vi "Destroy Broadcast Events.vi"(8 "error in (no error)":errorcluster) -> (0 "error out":errorcluster)   [LabVIEW 2015, in "Tool Module.lvlib"]
doc: "Destroy the broadcast events, even if there is an incoming error.\n\n<b>NOTE</b>: The contents of this VI are automatically generated and modified by the <b>Tools > Delacor > DQMH</b> utilities. Consider using those utilities instead of making your own modifications to this VI.\n_____\nBased on Delacor QMH Project Template 2.1.0.2."
uses:
  Tool Module.lvlib
panel:
  # "NOTE: The contents of this VI are automatically generated and modified by the Tools > Delacor > DQMH utilities. Consider using those utilities instead of making your own modifications to this VI."
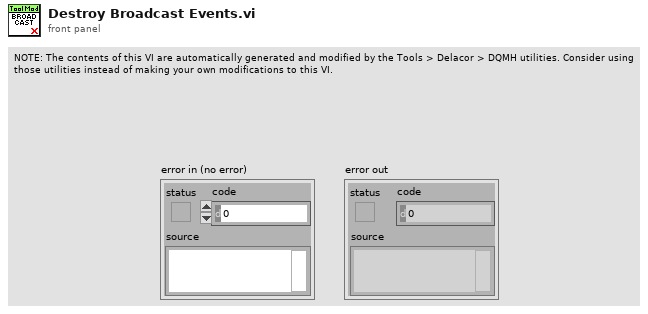
[diagram p1: front panel]
types:
  T1 = typedef "Tool Module.lvlib/Broadcast Events--cluster.ctl" = cluster{"Module Did Init":refnum<user-event>, "Status Updated":refnum<user-event>, "Error Reported":refnum<user-event>, "Module Did Stop":refnum<user-event>, "Update Module Execution Status":refnum<user-event>, "Send Status":refnum<user-event>, "Trigger":refnum<user-event>, "Connected":refnum<user-event>, "Read from File Rtn":refnum<user-event>, "Device Temperature":refnum<user-event>}
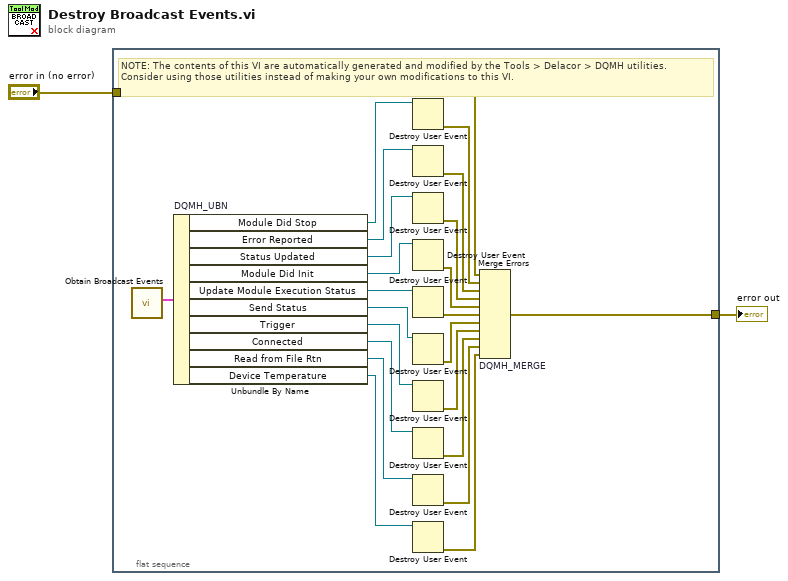
[diagram p0: block diagram]
diagram:
  n1 = flat-sequence {
    tunnel: [w24] -> w2
    tunnel: "error in (no error)" -> [w15]
    frame #0 {
      # "NOTE: The contents of this VI are automatically generated and modified by the Tools > Delacor > DQMH utilities. Consider using those utilities instead of making your own modifications to this VI."
      n2 = call "Obtain Broadcast Events.vi"() -> ("Tool Module Broadcast Events"=w23:T1)  [unwired: 10 in, 1 out]
      n3 = Unbundle By Name "DQMH_UBN"(w23) -> ("Module Did Stop"=w16:refnum<user-event>, "Error Reported"=w18:refnum<user-event>, "Status Updated"=w21:refnum<user-event>, "Module Did Init"=w22:refnum<user-event>, "Update Module Execution Status"=w13:refnum<user-event>, "Send Status"=w11:refnum<user-event>, "Trigger"=w9:refnum<user-event>, "Connected"=w7:refnum<user-event>, "Read from File Rtn"=w5:refnum<user-event>, "Device Temperature"=w3:refnum<user-event>)
      n4 = Destroy User Event(user event=w16) -> (error out=w17:errorcluster)  [unwired: 1 in]
      n5 = Destroy User Event(user event=w18) -> (error out=w19:errorcluster)  [unwired: 1 in]
      n6 = Destroy User Event(user event=w21) -> (error out=w20:errorcluster)  [unwired: 1 in]
      n7 = Destroy User Event(user event=w22) -> (error out=w25:errorcluster)  [unwired: 1 in]
      n8 = Destroy User Event(user event=w13) -> (error out=w14:errorcluster)  [unwired: 1 in]
      n9 = Destroy User Event(user event=w11) -> (error out=w12:errorcluster)  [unwired: 1 in]
      n10 = Destroy User Event(user event=w9) -> (error out=w10:errorcluster)  [unwired: 1 in]
      n11 = Destroy User Event(user event=w7) -> (error out=w8:errorcluster)  [unwired: 1 in]
      n12 = Destroy User Event(user event=w5) -> (error out=w6:errorcluster)  [unwired: 1 in]
      n13 = Destroy User Event(user event=w3) -> (error out=w4:errorcluster)  [unwired: 1 in]
      n14 = Merge Errors "DQMH_MERGE"(w15, w17, w19, w20, w25, w14, w12, w10, w8, w6, w4) -> (w24:errorcluster)
    }
  }
  "error out" <- w2
